vi "Host Globals.vi"() -> ()   [LabVIEW 2015]
uses:
  <vilib>/vision/Image Controls.llb/IMAQ Image.ctl
panel:
  in  "Image 2":T1
  in  "Image":T1
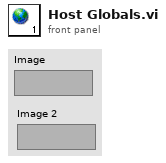
[diagram p1: front panel]
types:
  T1 = typedef "IMAQ Image.ctl" = refnum<image>
diagram:
